vi "JSON text to Variant (advanced).vi"(8 "error in (no error)":errorcluster, 9 "Data Type":variant, 10 "Offset":i32, 11 "JSON":string) -> (0 "error out":errorcluster, 1 "Variant out":variant)   [LabVIEW 2017, in "JSONtext.lvlib"]
doc: "Convert JSON to the Data Type entered, which may be a cluster or array."
uses:
  JSONtext.lvlib
  <vilib>/Utility/Data Type/Type Definitions/Data Type.ctl
  JSON Value Type.ctl
  support/Get String.vi
  support/Get LVObject.vi
  support/Get Timestamp.vi
  support/Get I32.vi
  support/Get I64.vi
  support/Get U32.vi
  support/Get U64.vi
  support/Get Boolean.vi
  support/Get DBL.vi
  support/Get SGL.vi
  support/quote and escape json string 2.vi
  Parsing/Advance past String.vi
  support/Format Error.vi
  support/Get Number Text.vi
  Parsing/NaN or null to Integer ERROR.vi
  Parsing/Advance past Number.vi
  Parsing/Parsing Error.vi
  <vilib>/Utility/error.llb/Error Cluster From Error Code.vi
  <vilib>/Utility/Data Type/Get Numeric Information.vi
  support/Unescape JSON string.vi
  support/Scan Timestamp.vi
  <vilib>/Utility/Data Type/Get Refnum Information.vi
  <vilib>/Utility/Data Type/NI_Data Type.lvlib
  <vilib>/JDP Science/JDP Science Common Utilities/JDP Utility.lvlib
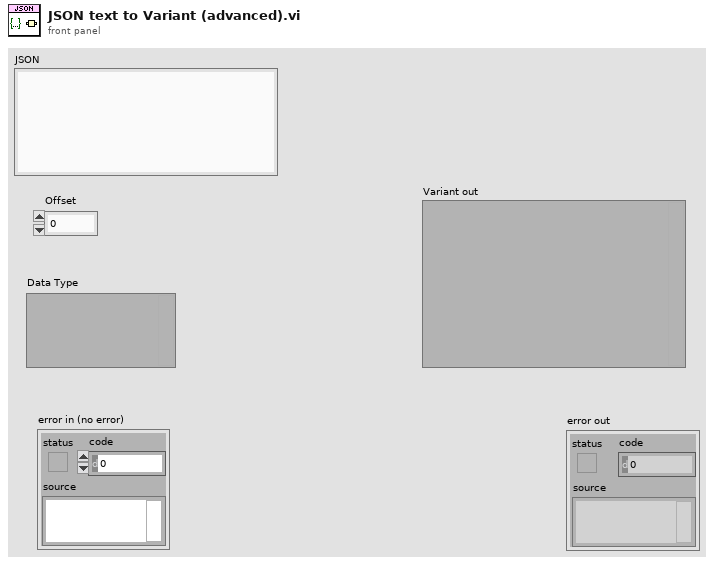
[diagram p1: front panel]
types:
  T1 = typedef "NI_Data Type.lvlib/Data Type.ctl" = enum8{"Invalid Type", "Void", "I8", "I16", "I32", "I64", "U8", "U16", "U32", "U64", "Single Float", "Double Float", "Extended Float", "Single Complex", "Double Complex", "Extended Complex", "Enum U8", "Enum U16", "Enum U32", "Enum U64", "Single Float With Unit", "Double Float With Unit", "Extended Float With Unit", "Single Complex with Unit", "Double Complex with Unit", "Extended Complex with Unit", "Boolean", "String", "Path", "Picture", "Tag", "Array", "Cluster", "Variant", "LV Variant", "Waveform", "Timestamp", "Digital Waveform", "Digital Data", "ExpressData", "Refnum", "External Data", "VI", "Poly VI", "LabVIEW Class Instance", "Fixed Point"}
  T2 = typedef "JSONtext.lvlib/Parsing State.ctl" = enum16{"Parser Error", "Object", "Array", "String", "Number/Other", "Leading Whitespace", "Object end", "Array end", "Value end"}
  T3 = typedef "JSONtext.lvlib/JSON Value Type.ctl" = enum16{"Not a JSON Value", "JSON Object", "JSON Array", "String", "Number", "true", "false", "null"}
  T4 = typedef "JSONtext.lvlib/Found Items.ctl" = cluster{"Item offset":i32, "Offset past Item":i32, "Name offset":i32, "Offset past Name":i32, "Found":bool, "Item Type":T2, "Item Index":i32}
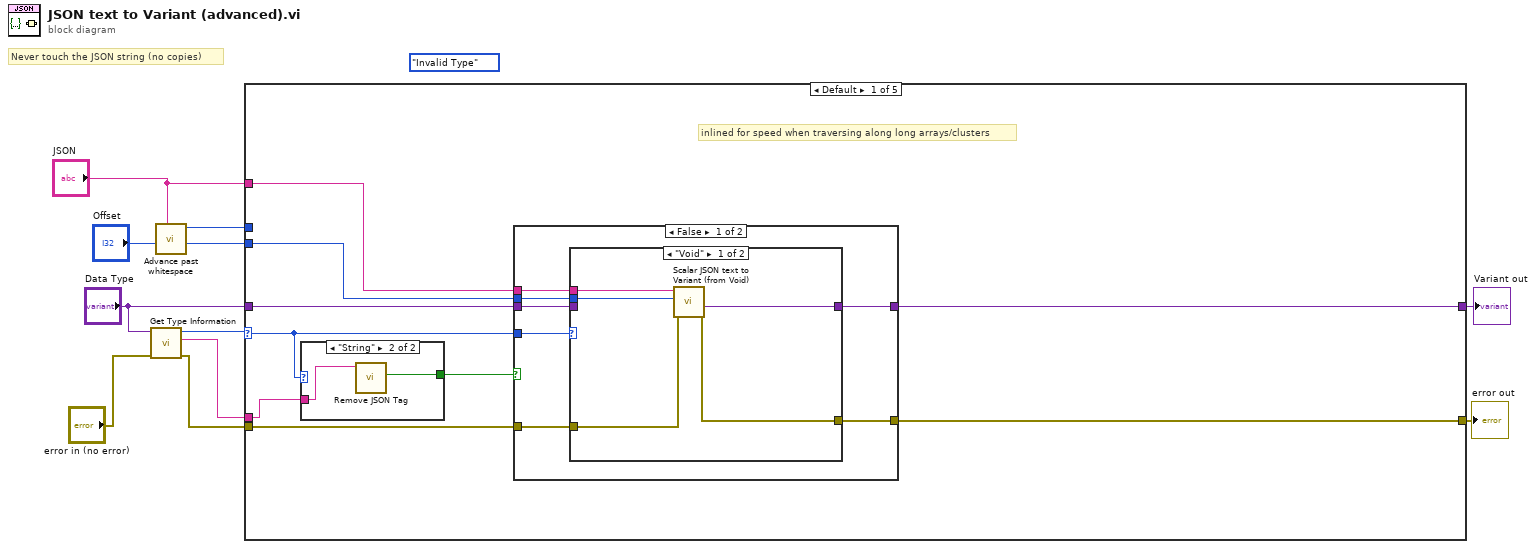
[diagram p0: block diagram]
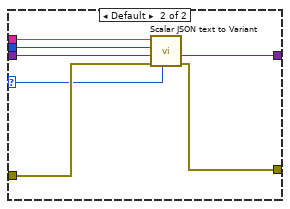
[diagram p2: hidden frame]
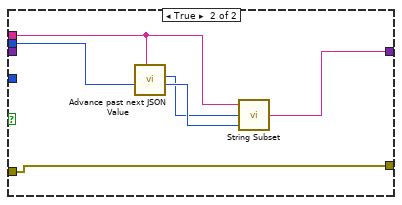
[diagram p3: hidden frame]
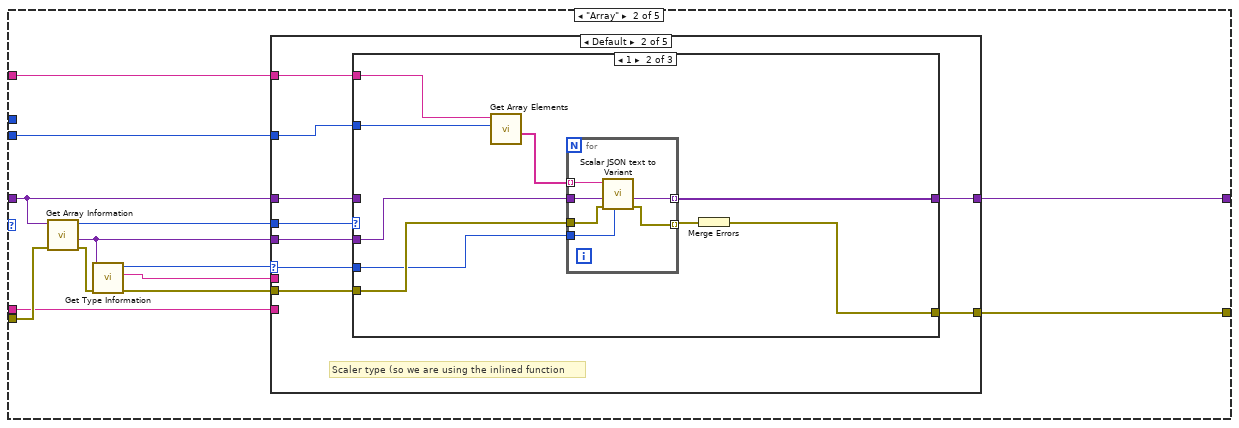
[diagram p5: hidden frame]
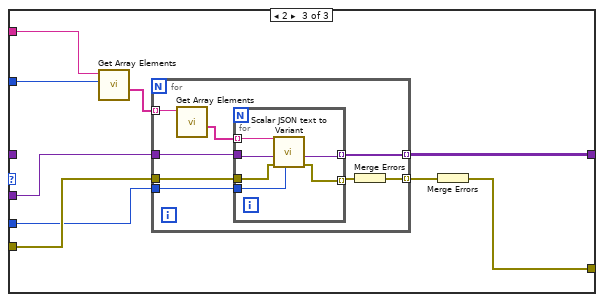
[diagram p8: hidden frame]
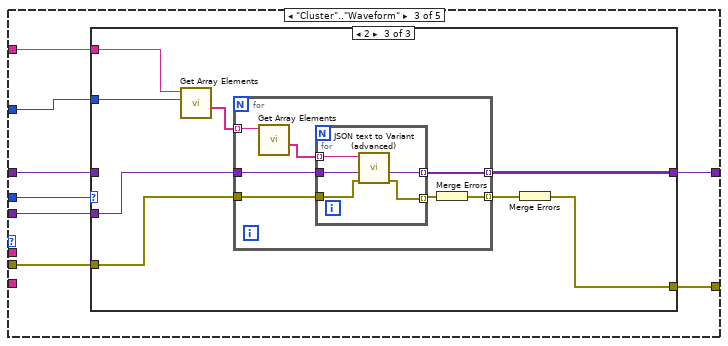
[diagram p9: hidden frame]
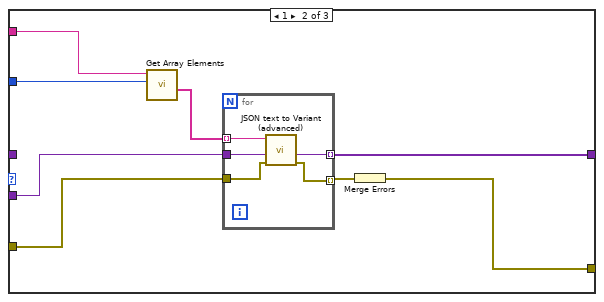
[diagram p11: hidden frame]
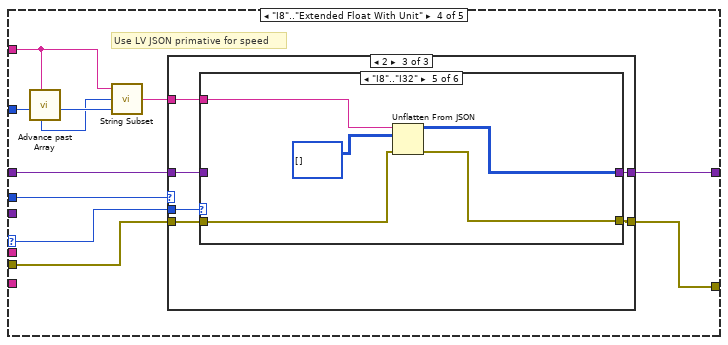
[diagram p12: hidden frame]
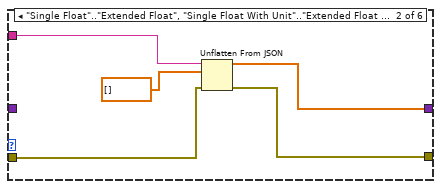
[diagram p15: hidden frame]
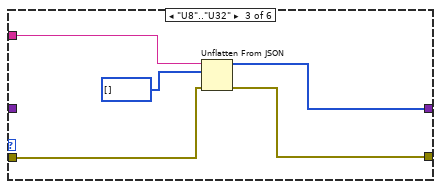
[diagram p16: hidden frame]
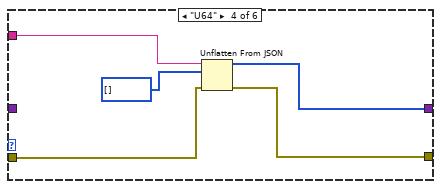
[diagram p17: hidden frame]
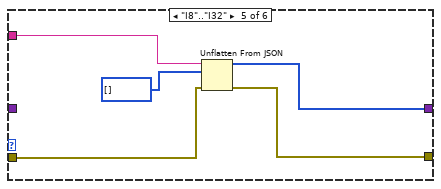
[diagram p18: hidden frame]
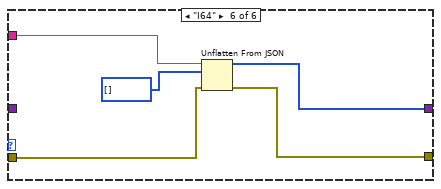
[diagram p19: hidden frame]
diagram:
  (unwired) Data_Type."Invalid Type" ("Type")
  # "Never touch the JSON string (no copies)"
  n1 = call <vilib>:"Get Type Information.vi"("error in (no error)"="error in (no error)", "Variant"="Data Type") -> ("error out"=w7:errorcluster, "Name"=w1:string, "Type"=w11:T1)  [unwired: 5 in, 2 out]
  n2 = call "Advance past whitespace.vi"("JSON"="JSON", "Offset"="Offset") -> ("Offset of first non-whitespace"=w4:i32, "Parser State"=w2:T2)  [unwired: 8 in]
  n3 = case shown="Default" w11 {
    selector: w11 -> [w13 _ _ _ _]
    tunnel: "Data Type" -> [w20 w53 w325 w338 w499]
    tunnel: "JSON" -> [w18 w51 w318 w330 w494]
    tunnel: [w15 w57 w315 w333 w491] -> w8
    tunnel: w7 -> [w16 w60 w324 w336 w498]
    tunnel: w4 -> [w17 w49 w317 w328 w493]
    tunnel: [w19 w56 w308 w334 w496] -> w6
    tunnel: w2 -> [_ _ _ _ _]
    tunnel: w1 -> [w14 w50 _ _ _]
    frame Default {
      # "inlined for speed when traversing along long arrays/clusters"
      n4 = case shown="\"String\"" w13 {
        tunnel: w14 -> [_ w47]
        tunnel: [_ w46] -> w12
        frame "Invalid Type", Default {
        }
        frame "String" {
          n5 = call "Remove JSON Tag.vi"("Name"=w47) -> ("tagged as JSON text"=w46:bool)  [unwired: 9 in, 1 out]
        }
      }
      n6 = case shown="False" w12 {
        tunnel: w20 -> [w27 _]
        tunnel: [w26 w41] -> w19
        tunnel: w18 -> [w25 w42]
        tunnel: w17 -> [w24 w45]
        tunnel: w16 -> [w23 w40]
        tunnel: [w22 w40] -> w15
        tunnel: w13 -> [w21 _]
        frame False {
          n7 = case shown="\"Void\"" w21 {
            selector: w21 -> [_ w33]
            tunnel: w27 -> [_ w39]
            tunnel: [w28 w38] -> w26
            tunnel: w25 -> [w31 w37]
            tunnel: w24 -> [w32 w36]
            tunnel: w23 -> [w30 w35]
            tunnel: [w29 w34] -> w22
            frame "Void" {
              n8 = call "Scalar JSON text to Variant (from Void).vi"("error in (no error)"=w30, "Offset"=w32, "JSON"=w31) -> ("error out"=w29:errorcluster, "Variant out"=w28:variant)  [unwired: 7 in]
            }
            frame Default {
              n9 = call "Scalar JSON text to Variant.vi"("Type"=w33, "error in (no error)"=w35, "Variant (Data Type)"=w39, "Offset"=w36, "JSON"=w37) -> ("error out"=w34:errorcluster, "Variant out"=w38:variant)  [unwired: 5 in]
            }
          }
        }
        frame True {
          n10 = call "Advance past next JSON Value.vi"("JSON"=w42, "Offset"=w45) -> ("Offset out"=w44:i32, "Value start"=w43:i32)  [unwired: 7 in, 1 out]
          n11 = call "String Subset.vi"("Offset past End"=w44, "Start offset"=w43, "JSON"=w42) -> ("substring"=w41:string)  [unwired: 2 in]
        }
      }
    }
    frame "Array" {
      n12 = call <vilib>:"Get Array Information.vi"("error in (no error)"=w60, "Variant"=w53) -> ("error out"=w59:errorcluster, "Array Element Data Type"=w52:variant, "Number of Dimensions"=w54:i32)  [unwired: 6 in, 1 out]
      n13 = call <vilib>:"Get Type Information.vi"("error in (no error)"=w59, "Variant"=w52) -> ("error out"=w58:errorcluster, "Name"=w48:string, "Type"=w55:T1)  [unwired: 5 in, 2 out]
      n14 = case shown="Default" w55 {
        selector: w55 -> [_ w63 _ w159 _]
        tunnel: w51 -> [_ w67 w115 w157 w245]
        tunnel: w58 -> [w61 w70 w118 w165 w244]
        tunnel: [w61 w71 w119 w164 w243] -> w57
        tunnel: [w62 w68 w116 w163 w242] -> w56
        tunnel: w54 -> [_ w66 w114 w162 w241]
        tunnel: w53 -> [w62 w65 w113 w161 w240]
        tunnel: w52 -> [_ w69 w117 _ _]
        tunnel: w49 -> [_ w64 w112 w156 w237]
        tunnel: w50 -> [_ _ _ _ w239]
        tunnel: w48 -> [_ _ _ _ w236]
        frame "Invalid Type" {
        }
        frame Default {
          # "Scaler type (so we are using the inlined function"
          n15 = case shown="1" w66 {
            tunnel: [w72 w81 w90] -> w71
            tunnel: w70 -> [w72 w80 w96]
            tunnel: w69 -> [_ w79 w95]
            tunnel: [w73 w77 w93] -> w68
            tunnel: w64 -> [_ w76 w92]
            tunnel: w67 -> [_ w75 w91]
            tunnel: w65 -> [w73 _ _]
            tunnel: w63 -> [_ w74 w89]
            frame 0, Default {
            }
            frame 1 {
              n16 = call "Get Array Elements.vi"("Offset"=w76, "JSON"=w75) -> ("<JSON>"=w78:string[])  [unwired: 7 in, 2 out]
              n17 = for {
                tunnel: w79 -> [w87]
                tunnel: w80 -> [w85]
                tunnel: [w84] -> w82 mode=indexing
                tunnel: [w86] -> w77 mode=indexing
                tunnel: w78 -> [w88] mode=indexing
                tunnel: w74 -> [w83]
                n18 = call "Scalar JSON text to Variant.vi"("Type"=w83, "error in (no error)"=w85, "Variant (Data Type)"=w87, "JSON"=w88) -> ("error out"=w84:errorcluster, "Variant out"=w86:variant)  [unwired: 6 in]
              }
              n19 = Merge Errors(w82) -> (w81:errorcluster)
            }
            frame 2 {
              n20 = call "Get Array Elements.vi"("Offset"=w92, "JSON"=w91) -> ("<JSON>"=w94:string[])  [unwired: 7 in, 2 out]
              n21 = for {
                tunnel: [w104] -> w97 mode=indexing
                tunnel: w96 -> [w103]
                tunnel: w95 -> [w102]
                tunnel: w94 -> [w100] mode=indexing
                tunnel: [w101] -> w93 mode=indexing
                tunnel: w89 -> [w98]
                n22 = call "Get Array Elements.vi"("JSON"=w100) -> ("<JSON>"=w99:string[])  [unwired: 8 in, 2 out]
                n23 = for {
                  tunnel: w102 -> [w107]
                  tunnel: w103 -> [w108]
                  tunnel: [w109] -> w105 mode=indexing
                  tunnel: [w110] -> w101 mode=indexing
                  tunnel: w99 -> [w111] mode=indexing
                  tunnel: w98 -> [w106]
                  n24 = call "Scalar JSON text to Variant.vi"("Type"=w106, "error in (no error)"=w108, "Variant (Data Type)"=w107, "JSON"=w111) -> ("error out"=w109:errorcluster, "Variant out"=w110:variant)  [unwired: 6 in]
                }
                n25 = Merge Errors(w105) -> (w104:errorcluster)
              }
              n26 = Merge Errors(w97) -> (w90:errorcluster)
            }
          }
        }
        frame "Cluster".."Waveform" {
          n27 = case shown="2" w114 {
            tunnel: [w120 w128 w135] -> w119
            tunnel: w118 -> [w120 w127 w141]
            tunnel: w117 -> [_ w126 w140]
            tunnel: [w121 w124 w138] -> w116
            tunnel: w112 -> [_ w123 w137]
            tunnel: w115 -> [_ w122 w136]
            tunnel: w113 -> [w121 _ _]
            frame 0, Default {
            }
            frame 1 {
              n28 = call "Get Array Elements.vi"("Offset"=w123, "JSON"=w122) -> ("<JSON>"=w125:string[])  [unwired: 7 in, 2 out]
              n29 = for {
                tunnel: w126 -> [w134]
                tunnel: w127 -> [w133]
                tunnel: [w132] -> w129 mode=indexing
                tunnel: [w131] -> w124 mode=indexing
                tunnel: w125 -> [w130] mode=indexing
                n30 = call "JSON text to Variant (advanced).vi"("error in (no error)"=w133, "Data Type"=w134, "JSON"=w130) -> ("error out"=w132:errorcluster, "Variant out"=w131:variant)  [unwired: 7 in]
              }
              n31 = Merge Errors(w129) -> (w128:errorcluster)
            }
            frame 2 {
              n32 = call "Get Array Elements.vi"("Offset"=w137, "JSON"=w136) -> ("<JSON>"=w139:string[])  [unwired: 7 in, 2 out]
              n33 = for {
                tunnel: [w148] -> w142 mode=indexing
                tunnel: w141 -> [w147]
                tunnel: w140 -> [w146]
                tunnel: w139 -> [w144] mode=indexing
                tunnel: [w145] -> w138 mode=indexing
                n34 = call "Get Array Elements.vi"("JSON"=w144) -> ("<JSON>"=w143:string[])  [unwired: 8 in, 2 out]
                n35 = for {
                  tunnel: w146 -> [w154]
                  tunnel: w147 -> [w153]
                  tunnel: [w152] -> w149 mode=indexing
                  tunnel: [w151] -> w145 mode=indexing
                  tunnel: w143 -> [w150] mode=indexing
                  n36 = call "JSON text to Variant (advanced).vi"("error in (no error)"=w153, "Data Type"=w154, "JSON"=w150) -> ("error out"=w152:errorcluster, "Variant out"=w151:variant)  [unwired: 7 in]
                }
                n37 = Merge Errors(w149) -> (w148:errorcluster)
              }
              n38 = Merge Errors(w142) -> (w135:errorcluster)
            }
          }
        }
        frame "I8".."Extended Float With Unit" {
          # "Use LV JSON primative for speed"
          n39 = call "Advance past Array.vi"("JSON"=w157, "Offset"=w156) -> ("Offset past Array"=w158:i32, "Array Start"=w155:i32)  [unwired: 7 in, 1 out]
          n40 = call "String Subset.vi"("Offset past End"=w158, "Start offset"=w155, "JSON"=w157) -> ("substring"=w160:string)  [unwired: 2 in]
          n41 = case shown="2" w162 {
            tunnel: w160 -> [_ w173 w206]
            tunnel: w165 -> [w166 w172 w205]
            tunnel: [w166 w171 w204] -> w164
            tunnel: [w167 w169 w202] -> w163
            tunnel: w161 -> [w167 w168 w201]
            tunnel: w159 -> [_ w170 w203]
            frame 0, Default {
            }
            frame 1 {
              n42 = case shown="\"Invalid Type\", Default" w170 {
                tunnel: w173 -> [_ w180 w185 w190 w195 w200]
                tunnel: w172 -> [w174 w178 w183 w188 w193 w198]
                tunnel: [w174 w177 w182 w187 w192 w197] -> w171
                tunnel: [w175 w176 w181 w186 w191 w196] -> w169
                tunnel: w168 -> [w175 _ _ _ _ _]
                frame "Invalid Type", Default {
                }
                frame "Single Float".."Extended Float", "Single Float With Unit".."Extended Float With Unit" {
                  n43 = Unflatten From JSON(JSON string=w180, type and defaults=dbl[] [], error in (no error)=w178) -> (value=w176:dbl[], error out=w177:errorcluster)  [unwired: 4 in]
                }
                frame "U8".."U32" {
                  n44 = Unflatten From JSON(JSON string=w185, type and defaults=u32[] [], error in (no error)=w183) -> (value=w181:u32[], error out=w182:errorcluster)  [unwired: 4 in]
                }
                frame "U64" {
                  n45 = Unflatten From JSON(JSON string=w190, type and defaults=u64[] [], error in (no error)=w188) -> (value=w186:u64[], error out=w187:errorcluster)  [unwired: 4 in]
                }
                frame "I8".."I32" {
                  n46 = Unflatten From JSON(JSON string=w195, type and defaults=i32[] [], error in (no error)=w193) -> (value=w191:i32[], error out=w192:errorcluster)  [unwired: 4 in]
                }
                frame "I64" {
                  n47 = Unflatten From JSON(JSON string=w200, type and defaults=i64[] [], error in (no error)=w198) -> (value=w196:i64[], error out=w197:errorcluster)  [unwired: 4 in]
                }
              }
            }
            frame 2 {
              n48 = case shown="\"I8\"..\"I32\"" w203 {
                tunnel: w206 -> [_ w213 w218 w223 w228 w233]
                tunnel: w205 -> [w207 w211 w216 w221 w226 w231]
                tunnel: [w207 w210 w215 w220 w225 w230] -> w204
                tunnel: [w208 w209 w214 w219 w224 w229] -> w202
                tunnel: w201 -> [w208 _ _ _ _ _]
                frame "Invalid Type", Default {
                }
                frame "Single Float".."Extended Float", "Single Float With Unit".."Extended Float With Unit" {
                  n49 = Unflatten From JSON(JSON string=w213, type and defaults=dbl[][] [], error in (no error)=w211) -> (value=w209:dbl[][], error out=w210:errorcluster)  [unwired: 4 in]
                }
                frame "U8".."U32" {
                  n50 = Unflatten From JSON(JSON string=w218, type and defaults=u32[][] [], error in (no error)=w216) -> (value=w214:u32[][], error out=w215:errorcluster)  [unwired: 4 in]
                }
                frame "U64" {
                  n51 = Unflatten From JSON(JSON string=w223, type and defaults=u64[][] [], error in (no error)=w221) -> (value=w219:u64[][], error out=w220:errorcluster)  [unwired: 4 in]
                }
                frame "I8".."I32" {
                  n52 = Unflatten From JSON(JSON string=w228, type and defaults=i32[][] [], error in (no error)=w226) -> (value=w224:i32[][], error out=w225:errorcluster)  [unwired: 4 in]
                }
                frame "I64" {
                  n53 = Unflatten From JSON(JSON string=w233, type and defaults=i64[][] [], error in (no error)=w231) -> (value=w229:i64[][], error out=w230:errorcluster)  [unwired: 4 in]
                }
              }
            }
          }
        }
        frame "String" {
          n54 = call "Remove JSON Tag.vi"("Name"=w236) -> ("tagged as JSON text"=w234:bool)  [unwired: 9 in, 1 out]
          n55 = call "Remove JSON Tag.vi"("Name"=w239) -> ("tagged as JSON text"=w238:bool)  [unwired: 9 in, 1 out]
          n56 = Or(x=w234, y=w238) -> (x .or. y?=w235:bool)
          n57 = case shown="False" w235 {
            tunnel: w245 -> [w252 w289]
            tunnel: w244 -> [w251 w288]
            tunnel: [w250 w287] -> w243
            tunnel: [w249 w286] -> w242
            tunnel: w241 -> [w248 w285]
            tunnel: w240 -> [w247 w284]
            tunnel: w237 -> [w246 w283]
            frame False {
              # "#ds issue #2 Can't use LV primative\nbecause it mishandles zero bytes."
              n58 = case shown="2" w248 {
                tunnel: w252 -> [_ w259 w267]
                tunnel: w251 -> [w253 w256 w268]
                tunnel: [w253 w257 w269] -> w250
                tunnel: [w254 w258 w270] -> w249
                tunnel: w247 -> [w254 _ _]
                tunnel: w246 -> [_ w255 w266]
                frame 0, Default {
                }
                frame 1 {
                  n59 = call "Get Array Elements.vi"("error in (no error)"=w256, "Offset"=w255, "JSON"=w259) -> ("error out"=w261:errorcluster, "<JSON>"=w260:string[])  [unwired: 6 in, 1 out]
                  n60 = for {
                    tunnel: w260 -> [w265] mode=indexing
                    tunnel: [w264] -> w258 mode=indexing
                    shift-right: [w263] -> w257
                    shift-left: w261 -> [w262]
                    n61 = call "Strip Quotes and Unescape.vi"("error in (no error)"=w262, "String"=w265) -> ("error out"=w263:errorcluster, "result string"=w264:string)  [unwired: 8 in]
                  }
                }
                frame 2 {
                  n62 = call "Get Array Elements.vi"("error in (no error)"=w268, "Offset"=w266, "JSON"=w267) -> ("error out"=w272:errorcluster, "<JSON>"=w271:string[])  [unwired: 6 in, 1 out]
                  n63 = for {
                    tunnel: w271 -> [w278] mode=indexing
                    tunnel: [w275] -> w270 mode=indexing
                    shift-right: [w274] -> w269
                    shift-left: w272 -> [w277]
                    n64 = call "Get Array Elements.vi"("error in (no error)"=w277, "JSON"=w278) -> ("error out"=w273:errorcluster, "<JSON>"=w276:string[])  [unwired: 7 in, 1 out]
                    n65 = for {
                      tunnel: w276 -> [w282] mode=indexing
                      tunnel: [w281] -> w275 mode=indexing
                      shift-right: [w280] -> w274
                      shift-left: w273 -> [w279]
                      n66 = call "Strip Quotes and Unescape.vi"("error in (no error)"=w279, "String"=w282) -> ("error out"=w280:errorcluster, "result string"=w281:string)  [unwired: 8 in]
                    }
                  }
                }
              }
            }
            frame True {
              # "JSON text"
              n67 = case shown="1" w285 {
                tunnel: w289 -> [_ w296 w298]
                tunnel: w288 -> [w290 w295 w299]
                tunnel: [w290 w294 w300] -> w287
                tunnel: [w291 w293 w301] -> w286
                tunnel: w284 -> [w291 _ _]
                tunnel: w283 -> [_ w292 w297]
                frame 0, Default {
                }
                frame 1 {
                  n68 = call "Get Array Elements.vi"("error in (no error)"=w295, "Offset"=w292, "JSON"=w296) -> ("error out"=w294:errorcluster, "<JSON>"=w293:string[])  [unwired: 6 in, 1 out]
                }
                frame 2 {
                  n69 = call "Get Array Elements.vi"("error in (no error)"=w299, "Offset"=w297, "JSON"=w298) -> ("error out"=w303:errorcluster, "<JSON>"=w302:string[])  [unwired: 6 in, 1 out]
                  n70 = for {
                    tunnel: w302 -> [w307] mode=indexing
                    tunnel: [w304] -> w301 mode=indexing
                    shift-right: [w305] -> w300
                    shift-left: w303 -> [w306]
                    n71 = call "Get Array Elements.vi"("error in (no error)"=w306, "JSON"=w307) -> ("error out"=w305:errorcluster, "<JSON>"=w304:string[])  [unwired: 7 in, 1 out]
                  }
                }
              }
            }
          }
        }
      }
    }
    frame "Waveform" {
      # "Attributes not supported"
      n72 = Variant To Data(error in=w324, type=waveform(dbl) {"t0"=timestamp(0 s since 1904-01-01), "dt"=1.0, "Y"=[]} ("waveform"), Variant=w325) -> (data=w322:waveform(dbl), error out=w316:errorcluster)
      n73 = Unbundle By Name(w322) -> ("t0"=w321:timestamp, "dt"=w320:dbl, "Y"=w319:dbl[])  [unwired: 1 out]
      n74 = Bundle("t0"=w321, "dt"=w320, "Y"=w319) -> (w313:cluster{"t0":timestamp, "dt":dbl, "Y":dbl[]})  [unwired: 1 in]
      n75 = call "JSON text to Variant (advanced).vi"("error in (no error)"=w316, "Data Type"=w313, "Offset"=w317, "JSON"=w318) -> ("error out"=w315:errorcluster, "Variant out"=w314:variant)  [unwired: 6 in]
      n76 = Variant To Data(type=w313, Variant=w314) -> (data=w312:cluster{"t0":timestamp, "dt":dbl, "Y":dbl[]})  [unwired: 1 in, 1 out]
      n77 = Unbundle By Name(w312) -> ("t0"=w311:timestamp, "dt"=w310:dbl, "Y"=w309:dbl[])
      n78 = Bundle By Name("t0"=w311, "dt"=w310, "Y"=w309) -> (w308:waveform(dbl))  [unwired: 1 in]
    }
    frame "Cluster" {
      n79 = Variant To Data(error in=w336, type=variant[] [], Variant=w338) -> (data=w326:variant[], error out=w332:errorcluster)
      n80 = Array Size(array=w326) -> (size(s)=w331:i32)
      n81 = case "Ragged Array?" shown="1" w331 {
        tunnel: w330 -> [_ w483]
        tunnel: [JSON_Value_Type."JSON Object" ("JSON Value Type") w482] -> w329
        tunnel: w328 -> [w473 w481]
        tunnel: [w473 w480] -> w327
        tunnel: w326 -> [_ w479]
        frame 0, Default {
        }
        frame 1 {
          n82 = Index Array(array=w479) -> (element=w478:variant)  [unwired: 1 in]
          n83 = call <vilib>:"Get Type Information.vi"("Variant"=w478) -> ("Type"=w477:T1)  [unwired: 6 in, 4 out]
          n84 = Equal?(x=Data_Type."Array", y=w477) -> (x = y?=w475:bool)
          n85 = case shown="True" w475 {
            tunnel: w483 -> [_ w489]
            tunnel: [JSON_Value_Type."JSON Object" ("JSON Value Type") w488] -> w482
            tunnel: w481 -> [w484 w487]
            tunnel: [w484 w486] -> w480
            frame False {
            }
            frame True {
              n86 = call "JSON type.vi"("Offset"=w487, "JSON"=w489) -> ("Item Offset"=w486:i32, "JSON Value Type"=w488:T3)  [unwired: 8 in]
            }
          }
        }
      }
      n87 = case shown="\"JSON Object\", Default" w329 {
        tunnel: [w349 w467] -> w335
        tunnel: [w348 w465] -> w333
        tunnel: w327 -> [w344 w469]
        tunnel: w332 -> [w343 w466]
        tunnel: w326 -> [w341 w472]
        tunnel: w330 -> [w340 w470]
        frame "JSON Object", Default {
          n88 = for {
            tunnel: w341 -> [w460] mode=indexing
            tunnel: w343 -> [w459]
            tunnel: [w458] -> w347 mode=indexing
            tunnel: [w456] -> w342 mode=indexing
            tunnel: [w457] -> w346 mode=indexing
            tunnel: [w454] -> w345 mode=indexing
            tunnel: [w450] -> w339
            i -> [w451]
            stop <- w450 stop-if-true
            n89 = call <vilib>:"Get Type Information.vi"("error in (no error)"=w459, "Variant"=w460) -> ("error out"=w458:errorcluster, "Name"=w455:string, "Type"=w456:T1)  [unwired: 5 in, 2 out]
            n90 = case shown="\"String\", \"Array\"" w456 {
              tunnel: w455 -> [w461 w464]
              tunnel: [_ w463] -> w457
              tunnel: [w461 w462] -> w453
              frame Default {
              }
              frame "String", "Array" {
                n91 = call "Remove JSON Tag.vi"("Name"=w464) -> ("tagged as JSON text"=w463:bool, "Name (tag stripped)"=w462:string)  [unwired: 9 in]
              }
            }
            n92 = Equal To 0?(x=w451) -> (x = 0?=w449:bool)
            n93 = Empty String/Path?(string/path=w453) -> (empty?=w452:bool)
            n94 = call "Quote and Escape JSON string.vi"("Plain Text"=w453) -> ("<JSON>"=w454:string)  [unwired: 10 in]
            n95 = And(x=w452, y=w449) -> (x .and. y?=w450:bool)
          }
          n96 = case shown="True" w339 {
            tunnel: [w362 w429] -> w349
            tunnel: [w361 w428] -> w348
            tunnel: w347 -> [w360 w432]
            tunnel: w346 -> [w358 _]
            tunnel: w345 -> [w357 _]
            tunnel: w344 -> [w356 w427]
            tunnel: w343 -> [w354 _]
            tunnel: w342 -> [w352 _]
            tunnel: w341 -> [w351 w431]
            tunnel: w340 -> [w350 w433]
            frame False {
              n97 = call "Find Object Item Locations by Names.vi"("Insertion point if not found"=TRUE, "Item Names <JSON>"=w357, "error in (no error)"=w354, "Object Offset"=w356, "JSON"=w350) -> ("error out"=w355:errorcluster, "Items"=w359:T4[])  [unwired: 5 in]
              n98 = for {
                tunnel: w351 -> [w374] mode=indexing
                tunnel: w350 -> [w373]
                tunnel: [w372] -> w363 mode=indexing
                tunnel: [w371] -> w362 mode=indexing
                tunnel: w360 -> [w370] mode=indexing
                tunnel: w352 -> [w369] mode=indexing
                tunnel: w359 -> [w368] mode=indexing
                tunnel: w358 -> [w364] mode=indexing
                n99 = Unbundle By Name(w368) -> ("Found"=w367:bool, "Item offset"=w366:i32, "Offset past Item"=w365:i32)
                n100 = case shown="True" w367 {
                  tunnel: w373 -> [_ w385]
                  tunnel: w366 -> [_ w384]
                  tunnel: w374 -> [w376 w383]
                  tunnel: [w376 w379] -> w371
                  tunnel: w370 -> [w375 w382]
                  tunnel: [w375 w381] -> w372
                  tunnel: w369 -> [_ w380]
                  tunnel: w365 -> [_ w377]
                  tunnel: w364 -> [_ w378]
                  frame False {
                  }
                  frame True {
                    n101 = case shown="True" w378 {
                      tunnel: w385 -> [w393 w414]
                      tunnel: w384 -> [w392 w413]
                      tunnel: w383 -> [w391 w407]
                      tunnel: w382 -> [w390 w409]
                      tunnel: [w389 w408] -> w381
                      tunnel: w380 -> [w386 w410]
                      tunnel: [w388 w411] -> w379
                      tunnel: w377 -> [_ w412]
                      frame False {
                        n102 = call "Is Scaler Type.vi"("Type"=w386) -> ("Scaler Type"=w387:bool)  [unwired: 2 in]
                        n103 = case shown="True" w387 {
                          tunnel: w393 -> [w400 w406]
                          tunnel: w392 -> [w399 w405]
                          tunnel: [w398 w404] -> w388
                          tunnel: w391 -> [w396 w403]
                          tunnel: w390 -> [w395 w402]
                          tunnel: [w397 w401] -> w389
                          tunnel: w386 -> [w394 _]
                          frame True {
                            n104 = call "Scalar JSON text to Variant.vi"("Type"=w394, "error in (no error)"=w395, "Variant (Data Type)"=w396, "Offset"=w399, "JSON"=w400) -> ("error out"=w397:errorcluster, "Variant out"=w398:variant)  [unwired: 5 in]
                          }
                          frame False {
                            n105 = call "JSON text to Variant (advanced).vi"("error in (no error)"=w402, "Data Type"=w403, "Offset"=w405, "JSON"=w406) -> ("error out"=w401:errorcluster, "Variant out"=w404:variant)  [unwired: 6 in]
                          }
                        }
                      }
                      frame True {
                        # "<JSON>"
                        n106 = case shown="\"Array\"" w410 {
                          tunnel: w414 -> [w420 w425]
                          tunnel: w413 -> [w419 w424]
                          tunnel: w412 -> [_ w423]
                          tunnel: [w416 w422] -> w411
                          tunnel: w409 -> [w417 w421]
                          tunnel: [w415 w421] -> w408
                          tunnel: w407 -> [w418 _]
                          frame "Array" {
                            n107 = call "JSON text to Variant (advanced).vi"("error in (no error)"=w417, "Data Type"=w418, "Offset"=w419, "JSON"=w420) -> ("error out"=w415:errorcluster, "Variant out"=w416:variant)  [unwired: 6 in]
                          }
                          frame "String", Default {
                            n108 = call "String Subset.vi"("Offset past End"=w423, "Start offset"=w424, "JSON"=w425) -> ("substring"=w422:string)  [unwired: 2 in]
                          }
                        }
                      }
                    }
                  }
                }
              }
              n109 = Merge Errors(w355, w363) -> (w361:errorcluster)
            }
            frame True {
              # "Unnamed cluster elements\n--> JSON Array"
              n110 = Merge Errors(w432) -> (w426:errorcluster)
              n111 = call "Get Array Elements.vi"("Offset"=w427, "JSON"=w433) -> ("<JSON>"=w430:string[])  [unwired: 7 in, 2 out]
              n112 = for {
                tunnel: w431 -> [w441] mode=indexing
                tunnel: w426 -> [w439]
                tunnel: [w438] -> w434 mode=indexing
                tunnel: [w440] -> w429 mode=indexing
                tunnel: w430 -> [w437]
                i -> [w435]
                n113 = Index Array(array=w437, index=w435) -> (element=w436:string)
                n114 = case shown="Default" w436 {
                  selector: w436 -> [_ w444]
                  tunnel: w441 -> [w443 w448]
                  tunnel: [w443 w447] -> w440
                  tunnel: w439 -> [w442 w446]
                  tunnel: [w442 w445] -> w438
                  frame "" {
                  }
                  frame Default {
                    n115 = call "JSON text to Variant (advanced).vi"("error in (no error)"=w446, "Data Type"=w448, "JSON"=w444) -> ("error out"=w445:errorcluster, "Variant out"=w447:variant)  [unwired: 7 in]
                  }
                }
              }
              n116 = Merge Errors(w434) -> (w428:errorcluster)
            }
          }
        }
        frame "JSON Array" {
          # "Let a JSON Array be valid for an Array as sole element in a Cluster, as this is a way of doing \"Ragged\" arrays in LabVIEW."
          n117 = Index Array(array=w472) -> (element=w471:variant)  [unwired: 1 in]
          n118 = call "JSON text to Variant (advanced).vi"("error in (no error)"=w466, "Data Type"=w471, "Offset"=w469, "JSON"=w470) -> ("error out"=w465:errorcluster, "Variant out"=w468:variant)  [unwired: 6 in]
          n119 = Build Array(w468) -> (w467:variant[])
        }
      }
      n120 = call <vilib>:"Array of Variants to Cluster.vi"("Array of Variants"=w335) -> ("Cluster of Variants"=w334:variant)  [unwired: 10 in]
    }
    frame "Variant", "LV Variant" {
      # "Unwrap and rewrap"
      n121 = Variant To Data(error in=w498, type=variant, Variant=w499) -> (data=w490:variant, error out=w495:errorcluster)
      n122 = call "JSON text to Variant (advanced).vi"("error in (no error)"=w495, "Data Type"=w490, "Offset"=w493, "JSON"=w494) -> ("error out"=w491:errorcluster, "Variant out"=w492:variant)  [unwired: 6 in]
      n123 = To Variant(anything=w492) -> (Variant=w496:variant)
    }
  }
  "Variant out" <- w6
  "error out" <- w8
